vi "Read output_.vi"(8 "error in":errorcluster, 11 "decideprojectfeatures in":refnum<class "DecideModuleFeatures.lvclass">) -> (0 "error out":errorcluster, 2 "output?":bool, 3 "decideprojectfeatures out":refnum<class "DecideModuleFeatures.lvclass">)   [LabVIEW 2013, in "DecideModuleFeatures.lvclass"]
uses:
  DecideModuleFeatures.lvclass
  DecideModuleFeatures.lvclass/DecideModuleFeatures.ctl
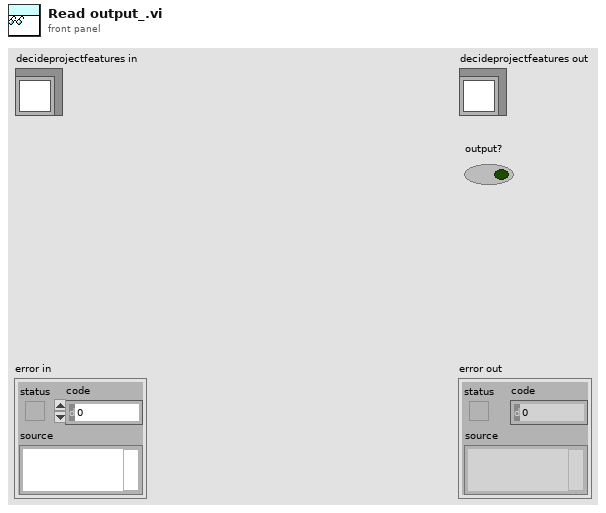
[diagram p1: front panel]
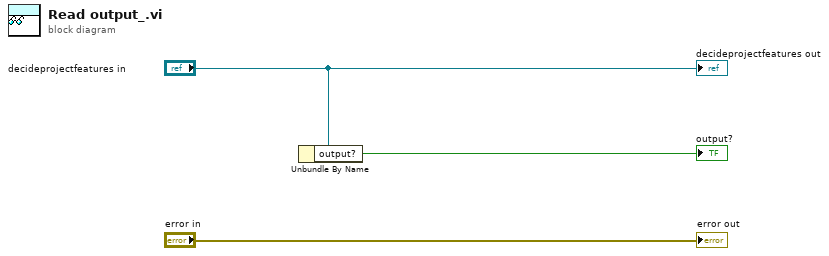
[diagram p0: block diagram]
diagram:
  n1 = Unbundle By Name("decideprojectfeatures in") -> ("output?"=→"output?":bool)
  "error out" <- "error in"
  "decideprojectfeatures out" <- "decideprojectfeatures in"
